vi "Set Test Log.vi"(10 "ITestLog.lvclass":refnum<class "Test Log.lvclass">, 11 "Model in":refnum<class "Model.lvclass">) -> (3 "Model out":refnum<class "Model.lvclass">)   [LabVIEW 2015, in "Model.lvclass"]
uses:
  Model.lvclass
  Test Log/Test Log/Test Log.lvclass
  Model.lvclass/Model.ctl
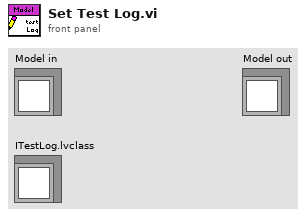
[diagram p1: front panel]
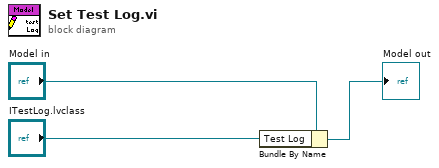
[diagram p0: block diagram]
diagram:
  n1 = Bundle By Name(cluster="Model in", "Test Log"="ITestLog.lvclass") -> (→"Model out":refnum<class "Model.lvclass">)
